vi "QueryStatus.vi"(8 "error in (no error)":errorcluster, 11 "ThorlabsLabJack in":refnum<class "ThorlabsLabJack.lvclass">) -> (0 "error out":errorcluster, 3 "ThorlabsLabJack out":refnum<class "ThorlabsLabJack.lvclass">)   [LabVIEW 2018, in "ThorlabsLabJack.lvlib" / "ThorlabsLabJack.lvclass"]
uses:
  ThorlabsLabJack.lvclass
  ThorlabsLabJack.lvclass/ThorlabsLabJack.ctl
  C:/AME Test Engineering/LabVIEW/PPLs/Axis/Thorlabs/Thorlabs.MotionControl.IntegratedStepperMotorsCLI.dll
  PPLs/Axis/Thorlabs/Thorlabs.MotionControl.IntegratedStepperMotorsCLI.dll
  C:/AME Test Engineering/LabVIEW/PPLs/Axis/DLLs/Thorlabs.MotionControl.GenericMotorCLI.dll
  PPLs/Axis/DLLs/Thorlabs.MotionControl.GenericMotorCLI.dll
  2d5f5b1d-1b6f-46fe-99cb-a2bc287bbde5.vi
  PPLs/Axis/Parent/Axis.lvlibp/Axis.lvclass
  C:/Projects/LWS_Base/trunk/LabVIEW/PPLs/Configuration/Axis.lvlibp/Axis.lvclass
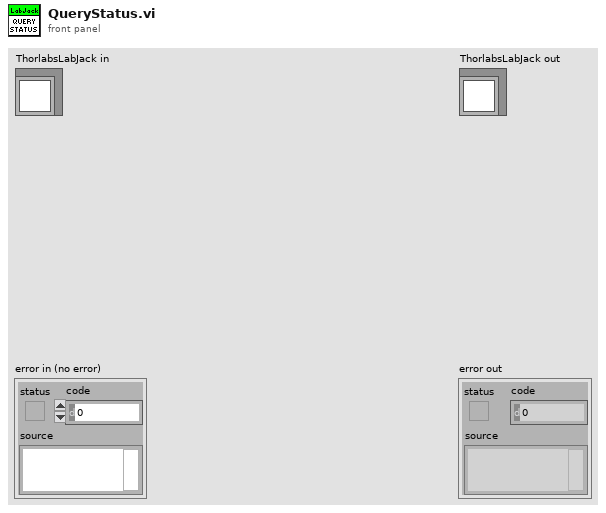
[diagram p1: front panel]
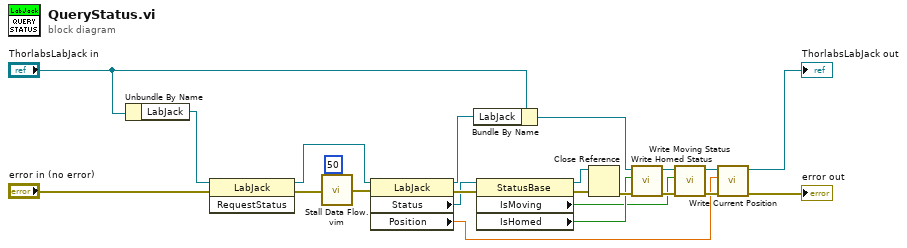
[diagram p0: block diagram]
diagram:
  n1 = Unbundle By Name("ThorlabsLabJack in") -> ("LabJack"=w22:refnum<k24>)
  n2 = invoke class="LabJack" method="RequestStatus"(reference=w22, error in="error in (no error)") -> (reference out=w17:refnum<k24>, error out=w20:errorcluster)  [unwired: 1 in, 1 out]
  n3 = call "Stall Data Flow.vim"("value in"=w20, "milliseconds to wait"=u32 50) -> ("value out"=w18:errorcluster)  [unwired: 1 out]
  n4 = property class="LabJack"(reference=w17, error in=w18) -> (reference out=w14:refnum<k24>, error out=w16:errorcluster, "Status"=w15:refnum<k24>, "Position"=w1:dbl)
  n5 = Bundle By Name(cluster="ThorlabsLabJack in", "LabJack"=w14) -> (w6:refnum<class "ThorlabsLabJack.lvclass">)
  n6 = property class="StatusBase"(reference=w15, error in=w16) -> (reference out=w4:refnum<k24>, error out=w11:errorcluster, "IsMoving"=w2:bool, "IsHomed"=w3:bool)
  n7 = Close Reference(reference=w4, error in (no error)=w11) -> (error out=w10:errorcluster)
  n8 = call "Write Homed Status.vi"("error in (no error)"=w10, "Homed?"=w3, "Axis in"=w6) -> ("error out"=w9:errorcluster, "Axis out"=w12:refnum<class "ThorlabsLabJack.lvclass">)  [unwired: 7 in]
  n9 = call "Write Moving Status.vi"("error in (no error)"=w9, "Moving?"=w2, "Axis in"=w12) -> ("error out"=w8:errorcluster, "Axis out"=w13:refnum<class "ThorlabsLabJack.lvclass">)  [unwired: 7 in]
  n10 = call "Write Current Position.vi"("error in"=w8, "Current Position"=w1, "Axis in"=w13) -> ("error out"=→"error out":errorcluster, "Axis out"=→"ThorlabsLabJack out":refnum<class "ThorlabsLabJack.lvclass">)  [unwired: 7 in]
